vi "email.vi"() -> ()   [LabVIEW 2020]
uses:
  <vilib>/smtpClient/Set Message Text.vi
  <vilib>/smtpClient/LabVIEWSMTPClient.lvlib
panel:
  in  "To":string
  in  "text message":string
  in  "subject":string
  in  "password":string
  in  "username":string
  in  "from":string
  in  "port":string
  in  "smtp ongoing":string
  # "Email using SMTP"
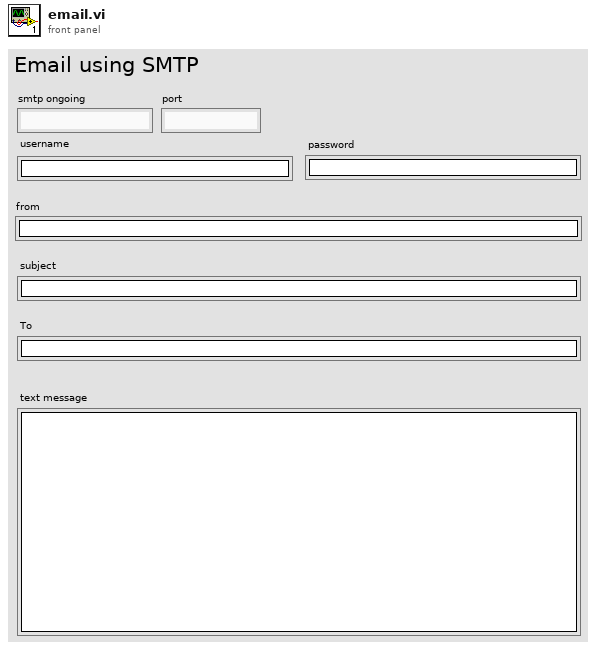
[diagram p1: front panel]
types:
  T1 = typedef "LabVIEWSMTPClient.lvlib/SmtpClientHandle.ctl" = refnum<k1>
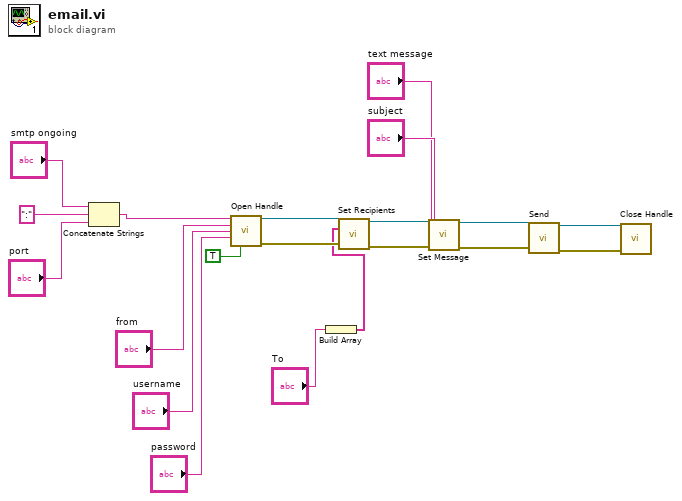
[diagram p0: block diagram]
diagram:
  n1 = Concatenate Strings("smtp ongoing", ":" ("string"), "port") -> (w12:string)
  n2 = call <vilib>:"Open Handle.vi"("server address"=w12, "from"="from", "username"="username", "password"="password", "use TLS (false)"=TRUE) -> ("handle out"=w20:T1, "error out"=w16:errorcluster)  [unwired: 9 in]
  n3 = Build Array("To") -> (w2:string[])
  n4 = call <vilib>:"Set Recipients.vi"("handle in"=w20, "to"=w2, "error in (no error)"=w16) -> ("handle out"=w19:T1, "error out"=w15:errorcluster)  [unwired: 11 in]
  n5 = call-poly <vilib>:"Set Message.vi"("handle in"=w19, "subject"="subject", "plain text message"="text message", "error in (no error)"=w15) -> ("handle out"=w18:T1, "error out"=w14:errorcluster)  [unwired: 10 in]
  n6 = call <vilib>:"Send.vi"("handle in"=w18, "error in (no error)"=w14) -> ("handle out"=w17:T1, "error out"=w13:errorcluster)  [unwired: 11 in, 1 out]
  n7 = call <vilib>:"Close Handle.vi"("handle in"=w17, "error in (no error)"=w13) -> ()  [unwired: 12 in, 2 out]
